vi "Unit Test LabJack.vi"() -> ()   [LabVIEW 2018]
uses:
  LWS_Base/trunk/LabVIEW/PPLs/Configuration/Axis.lvlibp/Custom Controls/Command.ctl
  ThorlabsLabJack.lvclass
  LWS_Base/trunk/LabVIEW/PPLs/Configuration/Axis.lvlibp/Custom Controls/Jog Direction.ctl
  LWS_Base/trunk/LabVIEW/PPLs/Configuration/Axis.lvlibp/Axis.lvclass
  LWS_Base/trunk/LabVIEW/PPLs/Configuration/Axis.lvlibp
  C:/Projects/LWS_Base/trunk/LabVIEW/PPLs/Configuration/Axis.lvlibp/Axis.lvclass
panel:
  in  "Stop":bool
  in  "Jog Forwad":bool
  in  "Jog Back":bool
  in  "Step Back":bool
  in  "Step Forward":bool
  out "Error Out":errorcluster
  in  "Error In":errorcluster
  out "Current Position":dbl
  in  "Value":dbl
  out "Homed?":bool
  out "Moving?":bool
  out "Home Success?":bool
  in  "Command":T1
  in  "Home":bool
  in  "SendCMD":bool
  in  "Device":string
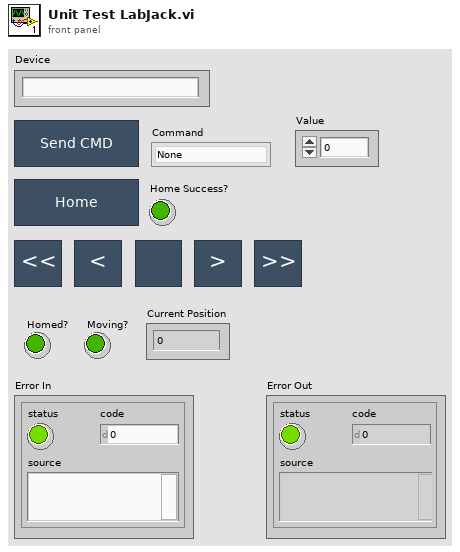
[diagram p1: front panel]
types:
  T1 = typedef "Axis.lvlibp/Command.ctl" = enum16{"None", "Home", "Renumber", "Move Absolute", "Move Relative", "Stop", "Set Run Speed", "Set Acceleration", "Set Run Current", "Set Home Offset", "Set Home Speed", "Query Current Position", "Load Defaults", "Query Status", "Lock Controls", "Unlock Controls", "Set Jog Step Size", "Set Jog Acceleration", "Set Jog Speed", "Query Homed Status", "Query Moving Status", "Reset"}
  T2 = typedef "Axis.lvlibp/Jog Direction.ctl" = enum16{"Forward", "Backward"}
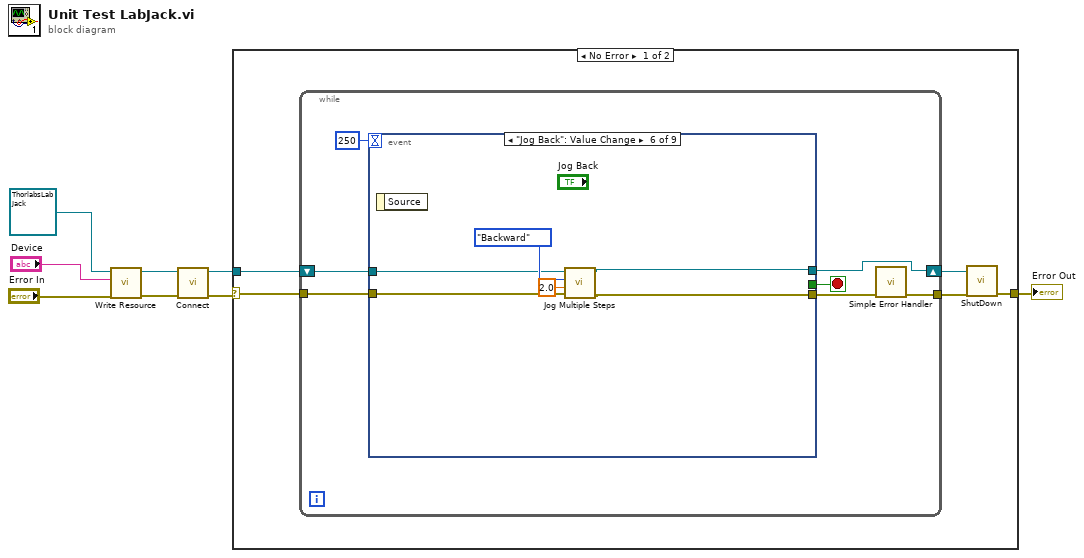
[diagram p0: block diagram]
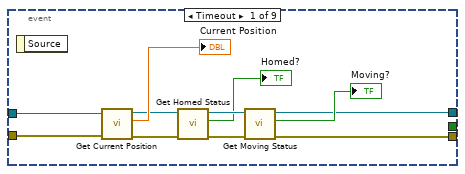
[diagram p2: hidden frame]
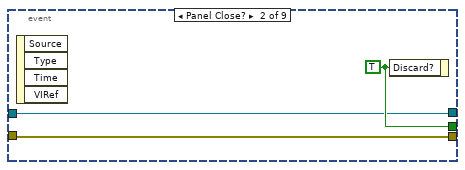
[diagram p3: hidden frame]
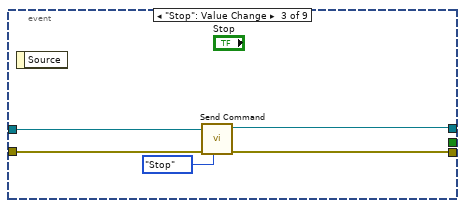
[diagram p4: hidden frame]
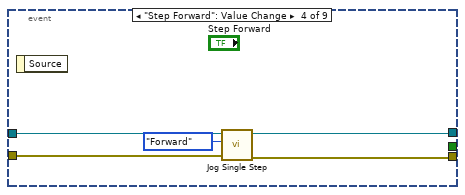
[diagram p5: hidden frame]
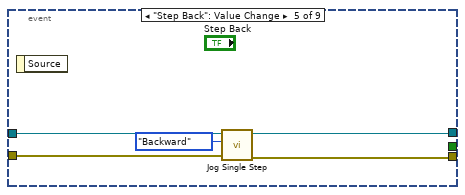
[diagram p6: hidden frame]
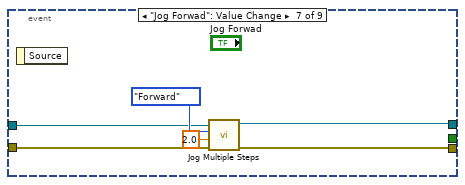
[diagram p7: hidden frame]
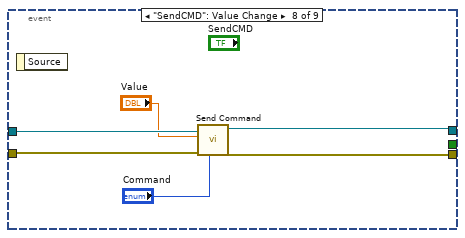
[diagram p8: hidden frame]
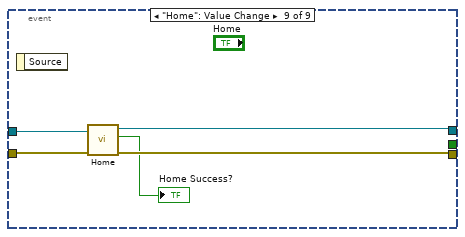
[diagram p9: hidden frame]
diagram:
  n1 = call "Write Resource.vi"("error in"="Error In", "Resource"="Device", "Axis in"=refnum<class "ThorlabsLabJack.lvclass"> refnum ("ThorlabsLabJack.lvlib:ThorlabsLabJack.lvclass")) -> ("error out"=w3:errorcluster, "Axis out"=w5:refnum<class "ThorlabsLabJack.lvclass">)  [unwired: 7 in]
  n2 = call-dynamic "Connect.vi"("error in"=w3, "ThorlabsLabJack in"=w5) -> ("error out"=w8:errorcluster, "ThorlabsLabJack out"=w7:refnum<class "ThorlabsLabJack.lvclass">)  [unwired: 8 in]
  n3 = case shown="No Error" w8 {
    selector: w8 -> [w12 w73]
    tunnel: w7 -> [w13 _]
    tunnel: [w9 w73] -> w1
    frame No Error {
      n4 = while {
        shift-right: [w17] -> w10
        shift-left: w13 -> [w19]
        tunnel: w12 -> [w18]
        tunnel: [w15] -> w11
        stop <- w14 stop-if-true
        n5 = event shown="[5] \"Jog Back\": Value Change" {
          selector: _ -> [_ _ _ _ _ _ _ _ _]
          dyn-events: _ -> [_ _ _ _ _ _ _ _ _]
          timeout: 250 -> [_ _ _ _ _ _ _ _ _]
          tunnel: w19 -> [w30 w33 w39 w44 w49 w54 w60 w67 w72]
          tunnel: w18 -> [w31 w32 w38 w43 w48 w53 w57 w64 w71]
          tunnel: [w22 w32 w35 w41 w46 w52 w58 w65 w69] -> w16
          tunnel: [w21 w33 w36 w42 w47 w51 w59 w66 w70] -> w17
          tunnel: [_ w34 _ _ _ _ _ _ _] -> w14
          event Timeout {
            n6 = event-data() -> ()  [unwired: 1 in, 1 out]
            n7 = call "Get Current Position.vi"("error in"=w31, "Axis in"=w30) -> ("error out"=w26:errorcluster, "Current Position"=→"Current Position":dbl, "Axis out"=w28:refnum<class "ThorlabsLabJack.lvclass">)  [unwired: 7 in]
            n8 = call "Get Homed Status.vi"("error in (no error)"=w26, "Axis in"=w28) -> ("error out"=w25:errorcluster, "Homed?"=→"Homed?":bool, "Axis out"=w27:refnum<class "ThorlabsLabJack.lvclass">)  [unwired: 7 in]
            n9 = call "Get Moving Status.vi"("error in (no error)"=w25, "Axis in"=w27) -> ("error out"=w22:errorcluster, "Moving?"=→"Moving?":bool, "Axis out"=w21:refnum<class "ThorlabsLabJack.lvclass">)  [unwired: 7 in]
          }
          event Panel Close? {
            w34 = TRUE ("Discard?")
            n10 = event-data() -> ()  [unwired: 1 in, 4 out]
            n11 = event-data("Discard?"=w34) -> ()  [unwired: 1 in, 1 out]
          }
          event "Stop": Value Change {
            n12 = event-data() -> ()  [unwired: 1 in, 1 out]
            n13 = call-dynamic "Send Command.vi"("Command"=Command."Stop", "error in"=w38, "ThorlabsLabJack in"=w39) -> ("error out"=w35:errorcluster, "ThorlabsLabJack out"=w36:refnum<class "ThorlabsLabJack.lvclass">)  [unwired: 7 in]
          }
          event "Step Forward": Value Change {
            n14 = event-data() -> ()  [unwired: 1 in, 1 out]
            n15 = call-dynamic "Jog Single Step.vi"("error in (no error)"=w43, "Jog Direction"=Jog_Direction."Forward", "ThorlabsLabJack in"=w44) -> ("error out"=w41:errorcluster, "ThorlabsLabJack out"=w42:refnum<class "ThorlabsLabJack.lvclass">)  [unwired: 7 in]
          }
          event "Step Back": Value Change {
            n16 = event-data() -> ()  [unwired: 1 in, 1 out]
            n17 = call-dynamic "Jog Single Step.vi"("error in (no error)"=w48, "Jog Direction"=Jog_Direction."Backward", "ThorlabsLabJack in"=w49) -> ("error out"=w46:errorcluster, "ThorlabsLabJack out"=w47:refnum<class "ThorlabsLabJack.lvclass">)  [unwired: 7 in]
          }
          event "Jog Back": Value Change {
            n18 = event-data() -> ()  [unwired: 1 in, 1 out]
            n19 = call-dynamic "Jog Multiple Steps.vi"("error in (no error)"=w53, "StepAmount"=2.0, "Jog Direction"=Jog_Direction."Backward", "ThorlabsLabJack in"=w54) -> ("error out"=w52:errorcluster, "ThorlabsLabJack out"=w51:refnum<class "ThorlabsLabJack.lvclass">)  [unwired: 6 in]
          }
          event "Jog Forwad": Value Change {
            n20 = event-data() -> ()  [unwired: 1 in, 1 out]
            n21 = call-dynamic "Jog Multiple Steps.vi"("error in (no error)"=w57, "StepAmount"=2.0, "Jog Direction"=Jog_Direction."Forward", "ThorlabsLabJack in"=w60) -> ("error out"=w58:errorcluster, "ThorlabsLabJack out"=w59:refnum<class "ThorlabsLabJack.lvclass">)  [unwired: 6 in]
          }
          event "SendCMD": Value Change {
            n22 = event-data() -> ()  [unwired: 1 in, 1 out]
            n23 = call-dynamic "Send Command.vi"("Command"="Command", "error in"=w64, "Value"="Value", "ThorlabsLabJack in"=w67) -> ("error out"=w65:errorcluster, "ThorlabsLabJack out"=w66:refnum<class "ThorlabsLabJack.lvclass">)  [unwired: 6 in]
          }
          event "Home": Value Change {
            n24 = event-data() -> ()  [unwired: 1 in, 1 out]
            n25 = call "Home.vi"("error in"=w71, "Axis in"=w72) -> ("error out"=w69:errorcluster, "Success?"=→"Home Success?":bool, "Axis out"=w70:refnum<class "ThorlabsLabJack.lvclass">)  [unwired: 7 in]
          }
        }
        n26 = call <vilib>:"Simple Error Handler.vi"("error in (no error)"=w16) -> ("error out"=w15:errorcluster)  [unwired: 4 in, 4 out]
      }
      n27 = call "ShutDown.vi"("error in"=w11, "Axis in"=w10) -> ("error out"=w9:errorcluster)  [unwired: 8 in, 1 out]
    }
    frame Error {
    }
  }
  "Error Out" <- w1
